vi "KeyControl.vi"(9 "Threshold":dbl, 10 "Channel weights":T1 {"W 8" scale=-10.0..10.0; "W 7" scale=-10.0..10.0; "W 6" scale=-10.0..10.0; "W 5" scale=-10.0..10.0; "W 4" scale=-10.0..10.0; "W 3" scale=-10.0..10.0; "W 2" scale=-10.0..10.0; "W 1" scale=-10.0..10.0}, 11 "Input":dbl[](array[numeric])) -> (1 "x > y?":bool, 3 "sum":dbl)   [LabVIEW 2023]
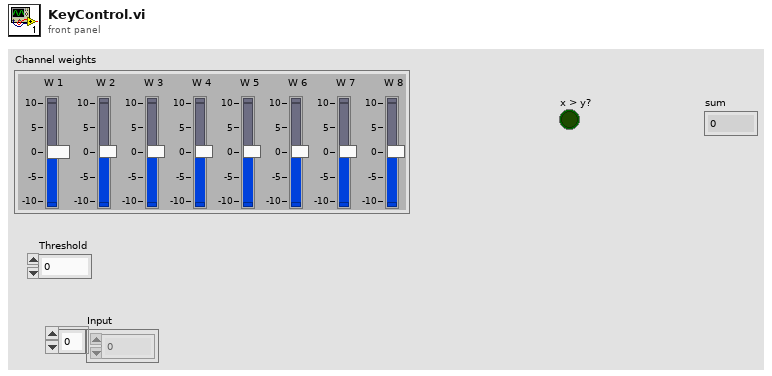
[diagram p1: front panel]
types:
  T1 = cluster{"W 1":dbl, "W 2":dbl, "W 3":dbl, "W 4":dbl, "W 5":dbl, "W 6":dbl, "W 7":dbl, "W 8":dbl}
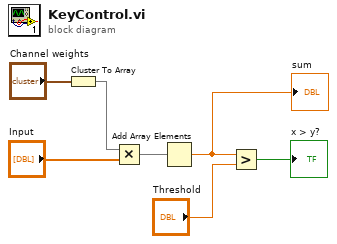
[diagram p0: block diagram]
diagram:
  n1 = Cluster To Array(cluster="Channel weights") -> (array=w2:dbl[])
  n2 = Multiply(x=w2, y="Input") -> (x*y=w6:dbl[])
  n3 = Add Array Elements(numeric array=w6) -> (sum=w3:dbl)
  "sum" <- w3
  n4 = Greater?(x=w3, y="Threshold") -> (0:→"x > y?":bool)
